vi "Get nixnet_grpc_CreateSessionMode for Value.vi"(8 "error in (no error)":errorcluster, 10 "proto enum value":i32, 11 "gRPC ID":T1) -> (0 "error out":errorcluster, 2 "labview enum value":u32, 3 "gRPC ID Out":T1)   [LabVIEW 2025, in "grpc-xnet_client.lvlib"]
uses:
  grpc-xnet_client.lvlib
  <vilib>/gRPC/LabVIEW gRPC Library/Shared/grpcId.ctl
  <vilib>/gRPC/LabVIEW gRPC Library/Shared/TranslateGrpcError.vi
  <vilib>/gRPC/LabVIEW gRPC Library/Server API/Server/Get Server DLL Path.vi
  <vilib>/Utility/error.llb/Error Cluster From Error Code.vi
  <vilib>/gRPC/LabVIEW gRPC Library/grpc-lvsupport-release.lvlib
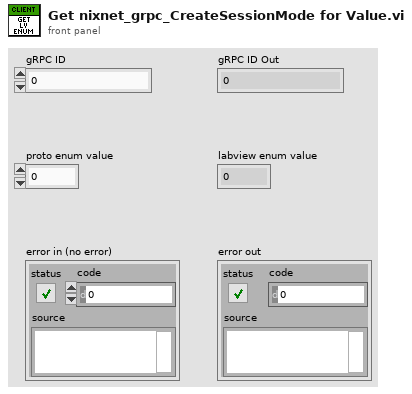
[diagram p1: front panel]
types:
  T1 = typedef "grpc-lvsupport-release.lvlib/grpcId.ctl" = u64
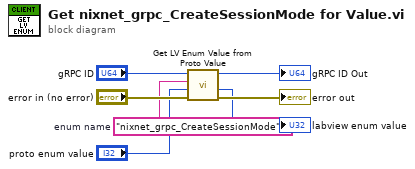
[diagram p0: block diagram]
diagram:
  w3 = "nixnet_grpc_CreateSessionMode"  # enum name
  n1 = call <vilib>:"Get LV Enum Value from Proto Value.vi"("error in"="error in (no error)", "proto enum value"="proto enum value", "enum name"=w3, "gRPCid in"="gRPC ID") -> ("error out"=→"error out":errorcluster, "labview enum value"=→"labview enum value":u32, "gRPCid out"=→"gRPC ID Out":T1)  [unwired: 5 in]
